vi "Mode of Operation Value Change.vi"(8 "error in (no error)":errorcluster, 10 "Mode of Operation":T1, 11 "Door Controller in":refnum<class "Door Controller.lvclass">) -> (0 "error out":errorcluster, 3 "Door Controller out":refnum<class "Door Controller.lvclass">)   [LabVIEW 2020, in "Door Controller.lvlib" / "Door Controller.lvclass"]
uses:
  Door Controller.lvclass
  Door Interlocks/Mode of Operation.ctl
  Door Controller.lvclass/Door Controller.ctl
  Door Interlocks/Door Interlocks.lvclass
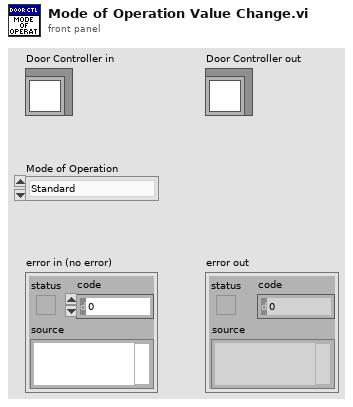
[diagram p1: front panel]
types:
  T1 = typedef "Door Interlocks.lvclass/Mode of Operation.ctl" = enum16{"Standard", "Interlock Override"}
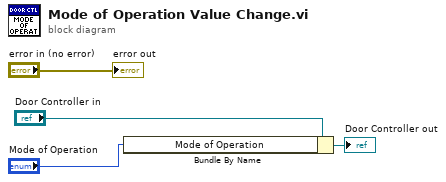
[diagram p0: block diagram]
diagram:
  n1 = Bundle By Name(cluster="Door Controller in", "Mode of Operation"="Mode of Operation") -> (→"Door Controller out":refnum<class "Door Controller.lvclass">)
  "error out" <- "error in (no error)"
